vi "数字输入_连续(端口).vi"() -> ()   [LabVIEW 2013]
doc: "This example demonstrates how to read values from a digital input port."
uses:
  <userlib>/ArtDAQ/_SubVI/ArtDAQ_CreateDIChan.vi
  <userlib>/ArtDAQ/_SubVI/ArtDAQ_CfgSampClkTiming.vi
  <userlib>/ArtDAQ/_SubVI/ArtDAQ_CfgDigEdgeStartTrig.vi
  <userlib>/ArtDAQ/_SubVI/ArtDAQ_Read Digital Bool(Port) 1Chan NSamp.vi
panel:
  out "数据":bool[][](array[boolean])
  out "错误输出":errorcluster
  in  "?":enum32{"No Trigger", "Digital Start"}(tab)
  in  "触发方向":i32(ring)=10280 items=["上升"=10280, "下降"=10171]
  in  "触发源":string="/Dev1/PFI0"
  in  "每通道采样数":i32=100
  in  "采样速率":dbl=1000.0
  in  "时钟源":string="/Dev1/PFI0"
  in  "?":bool
  in  "端口":string="Dev1/port0"
  # "通道属性"
  # "定时"
  # "触发"
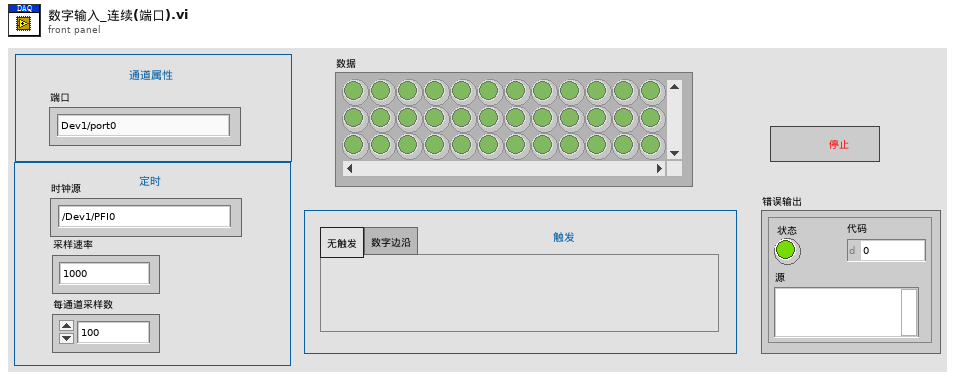
[diagram p1: front panel]
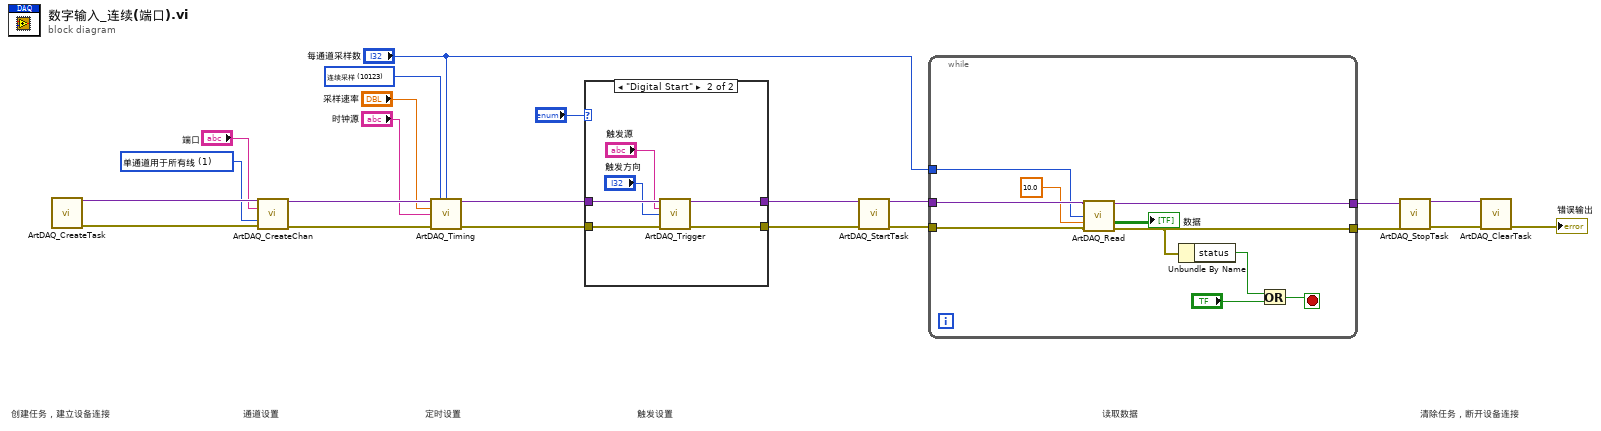
[diagram p0: block diagram]
diagram:
  w8 = 10123 items=["有限点采样"=10178, "连续采样"=10123] ("采样模式")
  w13 = 1 items=["单通道用于单条线", "单通道用于所有线"] ("Line Grouping")
  # "清除任务，断开设备连接"
  # "读取数据"
  # "触发设置"
  # "定时设置"
  # "通道设置"
  # "创建任务，建立设备连接"
  n1 = call <userlib>:"ArtDAQ_CreateTask.vi"() -> ("任务句柄"=w22:variant, "错误输出"=w21:errorcluster)  [unwired: 14 in]
  n2 = call-poly <userlib>:"ArtDAQ_CreateChan.vi"("任务句柄"=w22, "线"="端口", "线分组"=w13, "错误输入"=w21) -> ("任务句柄"=w11:variant, "错误输出"=w12:errorcluster)  [unwired: 10 in]
  n3 = call-poly <userlib>:"ArtDAQ_Timing.vi"("任务句柄"=w11, "采样模式"=w8, "每通道采样数"="每通道采样数", "采样率"="采样速率", "源"="时钟源", "错误输入"=w12) -> ("任务句柄"=w6:variant, "错误输出"=w5:errorcluster)  [unwired: 8 in]
  n4 = case shown="\"Digital Start\"" "?" {
    tunnel: w6 -> [w24 w30]
    tunnel: w5 -> [w23 w29]
    tunnel: [w24 w28] -> w4
    tunnel: [w23 w27] -> w3
    frame "No Trigger", Default {
    }
    frame "Digital Start" {
      n5 = call-poly <userlib>:"ArtDAQ_Trigger.vi"("任务句柄"=w30, "触发源"="触发源", "边沿"="触发方向", "错误输入"=w29) -> ("任务句柄"=w28:variant, "错误输出"=w27:errorcluster)  [unwired: 10 in]
    }
  }
  n6 = call <userlib>:"ArtDAQ_StartTask.vi"("任务句柄"=w4, "错误输入"=w3) -> ("任务句柄"=w20:variant, "错误输出"=w19:errorcluster)  [unwired: 12 in]
  n7 = while {
    tunnel: w20 -> [w40]
    tunnel: w19 -> [w39]
    tunnel: [w38] -> w18
    tunnel: [w36] -> w17
    tunnel: "每通道采样数" -> [w31]
    stop <- w33 stop-if-true
    n8 = call-poly <userlib>:"ArtDAQ_Read.vi"("任务句柄"=w40, "每通道采样数"=w31, "超时s"=10.0 ("Timeout"), "错误输入"=w39) -> ("任务句柄"=w38:variant, "数据"=→"数据":bool[][], "错误输出"=w36:errorcluster)  [unwired: 9 in]
    n9 = Unbundle By Name(w36) -> ("status"=w35:bool)
    n10 = Or(x=w35, y="?") -> (x .or. y?=w33:bool)
  }
  n11 = call <userlib>:"ArtDAQ_StopTask.vi"("任务句柄"=w18, "错误输入"=w17) -> ("任务句柄"=w15:variant, "错误输出"=w16:errorcluster)  [unwired: 12 in]
  n12 = call <userlib>:"ArtDAQ_ClearTask.vi"("任务句柄"=w15, "错误输入"=w16) -> ("错误输出"=→"错误输出":errorcluster)  [unwired: 13 in]
